vi "LVClasse_Phase ctor from HasoSlopes.vi"(0 "Phase (const)":refnum<class "Phase.lvclass">, 1 "Number of coefficients":u8, 5 "HasoSlopes":refnum<class "HasoSlopes.lvclass">, 7 "TypePhase":T1, 9 "Filter":u8[](array[numeric]), 11 "error in (no error)":errorcluster) -> (4 "Phase (new)":refnum<class "Phase.lvclass">, 6 "HasoSlopes (dup)":refnum<class "HasoSlopes.lvclass">, 15 "error out":errorcluster)   [LabVIEW 2020, in "Phase.lvclass"]
doc: "<B>PhaseIn</B> : Constant Pointer to Phase object. Phase sampling steps unit is um.\n<B>PhaseOut</B> : Constant Pointer to Phase object. Phase sampling steps unit is um.\n<B>HasoSlopes</B> : HasoSlopes object.\n<B>m_type</B> : E_COMPUTEPHASESET_T Phase reconstruction mode (Modal Legendre, Modal Zernike\n or Zonal only)\n<B>filter</B> : Array of aberrations to filter Filter must be a 5 elements array\n<B>nb_coeffs</B> : Optional number of coefficients to use for reconstruction. This parameters is\n mandatory if case Phase reconstruction mode is Modal Legendre or Modal\n Zernike, This parameters is ignored in reconstruction mode Zonal."
uses:
  Phase.lvclass
  WavefrontReconstructionMode.ctl
  HasoSlopes.lvclass
  Handle creation.ctl
  Phase.lvclass/Phase.ctl
  LVClass_HasoSlopes Read HasoSlopes _ property.vi
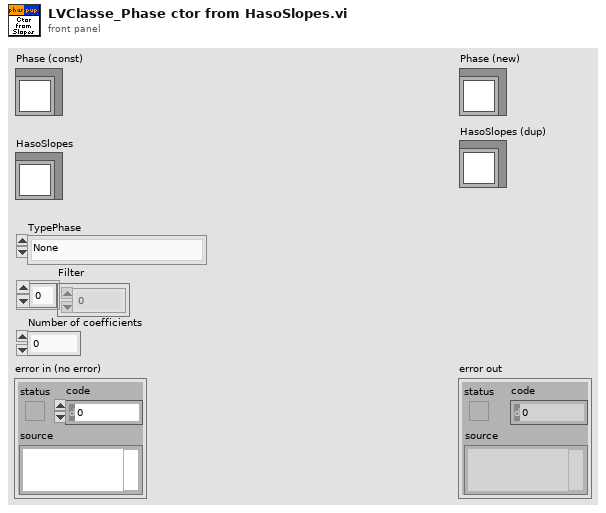
[diagram p1: front panel]
types:
  T1 = typedef "WavefrontReconstructionMode.ctl" = enum16{"None", "Modal_Legendre", "Modal_Zernike", "Zonal", "Modal_Zonal_Zernike", "Modal_Zonal_Legendre"}
  T2 = typedef "Handle creation.ctl" = enum16{"By ctor", "By write function"}
  T3 = typedef "ClassID.ctl" = i64
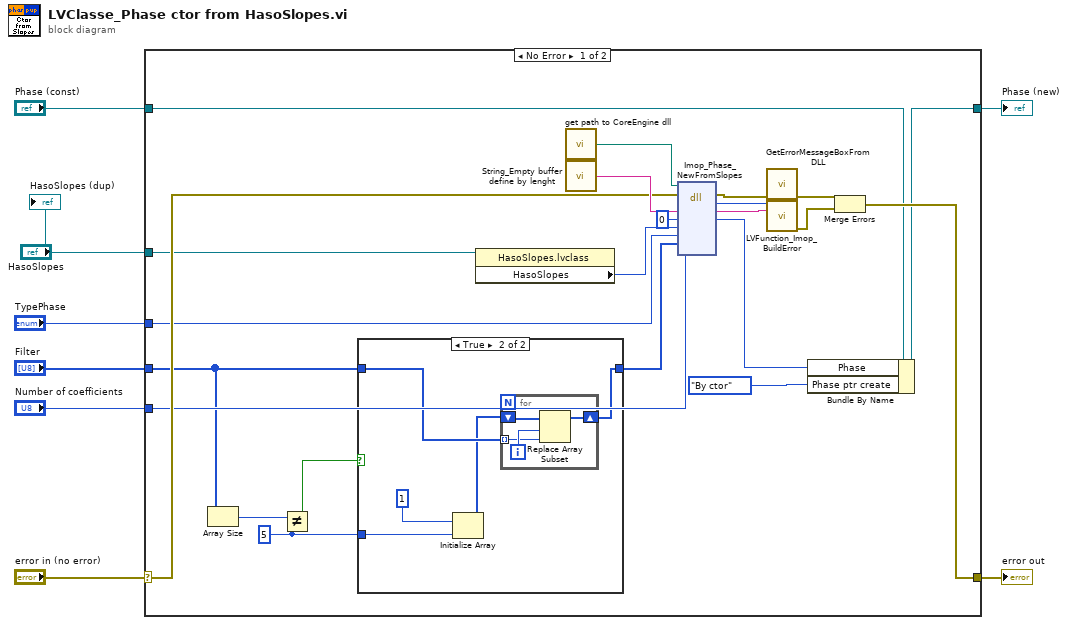
[diagram p0: block diagram]
diagram:
  n1 = case shown="No Error" "error in (no error)" {
    selector: "error in (no error)" -> [w24 w43]
    tunnel: [w23 w43] -> w7
    tunnel: [w17 w42] -> w5
    tunnel: "Phase (const)" -> [w18 w42]
    tunnel: "HasoSlopes" -> [w22 _]
    tunnel: "Filter" -> [w11 _]
    tunnel: "Number of coefficients" -> [w20 _]
    tunnel: "TypePhase" -> [w19 _]
    frame No Error {
      w10 = 5 ("y")
      n2 = Array Size(array=w11) -> (size(s)=w13:i32)
      n3 = Not Equal?(x=w13, y=w10) -> (x != y?=w12:bool)
      n4 = case shown="True" w12 {
        tunnel: w11 -> [w32 w35]
        tunnel: w10 -> [_ w37]
        tunnel: [w32 w33] -> w9
        frame False {
        }
        frame True {
          n5 = Initialize Array(1 ("Numeric"), w37) -> (w34:i32[])
          n6 = for {
            shift-right: [w40] -> w33
            shift-left: w34 -> [w41]
            tunnel: w35 -> [w38] mode=indexing
            i -> [w39]
            n7 = Replace Array Subset(array=w41, new element=w38, index=w39) -> (w40:i32[])
          }
        }
      }
      n8 = property class="HasoSlopes.lvclass"(reference=w22) -> ("HasoSlopes"=w21:T3)  [unwired: 1 in, 2 out]
      n9 = call "get path to CoreEngine dll.vi"() -> ("path to wavekit library"=w28:path)  [unwired: 14 in, 1 out]
      n10 = call "String_Empty buffer define by lenght.vi"() -> ("Empty buffer"=w29:string)  [unwired: 1 in]
      n11 = dll-call lib="D:/FLE/0.Code/CoreEngine4_Suite/LV2011_interface/DLLs/c_interface_vc100.dll" fn="Imop_Phase_NewFromSlopes"(path in=w28, error in=w24, "message"=w29, "Phase"=0, "HasoSlopes"=w21, "m-type"=w19, "Filter"=w9, "Coefficients"=w20) -> (error out=w27:errorcluster, "return type"=w31:i32, "message"=w30:string, "Phase"=w16:i64)  [unwired: 5 in, 1 out]
      n12 = call "GetErrorMessageBoxFromDLL.vi"("error IN"=w27) -> ("error OUT"=w26:errorcluster)  [unwired: 10 in]
      n13 = call "LVFunction_Imop_BuildError.vi"("code"=w31, "String to Prepend to source (\"\")"=w30) -> ("error out"=w25:errorcluster)  [unwired: 13 in]
      n14 = Bundle By Name(cluster=w18, "Phase"=w16, "Phase ptr create"=Handle_creation."By ctor") -> (w17:refnum<class "Phase.lvclass">)
      n15 = Merge Errors(w26, w25) -> (w23:errorcluster)
    }
    frame Error {
    }
  }
  "error out" <- w7
  "Phase (new)" <- w5
  "HasoSlopes (dup)" <- "HasoSlopes"
